vi "printDaqChannel.vi"(8 "error in":errorcluster, 9 "Indent":i32, 10 "TreeRef":refnum<vi>, 11 "baseObject in":refnum<class "IBaseObject.lvclass">) -> (0 "error out":errorcluster, 3 "baseObject out":refnum<class "IBaseObject.lvclass">)   [LabVIEW 2022 SP3, in "openDAQ.lvlib" / "daqUtils.lvlib" / "Tree.lvlib"]
uses:
  Tree.lvlib
  IBaseObject/IBaseObject.lvclass
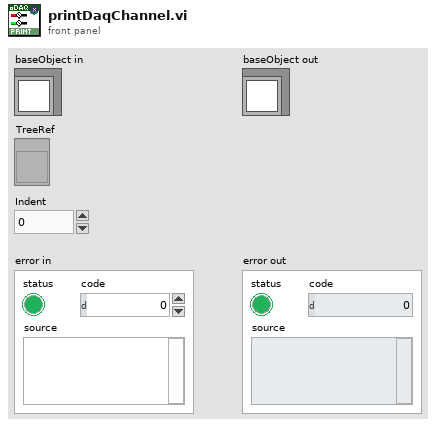
[diagram p1: front panel]
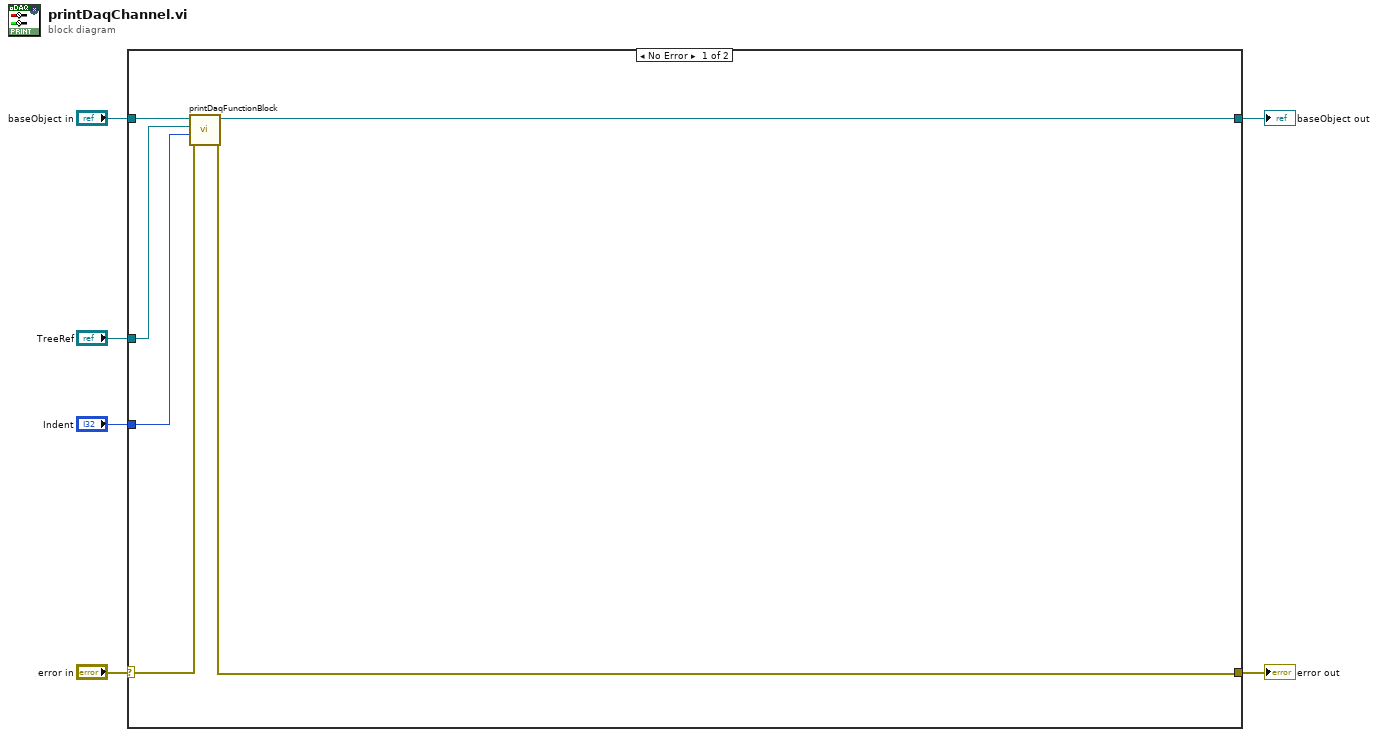
[diagram p0: block diagram]
diagram:
  n1 = case shown="No Error" "error in" {
    selector: "error in" -> [w11 w14]
    tunnel: "baseObject in" -> [w12 w13]
    tunnel: "Indent" -> [w7 _]
    tunnel: "TreeRef" -> [w8 _]
    tunnel: [w9 w14] -> w2
    tunnel: [w10 w13] -> w1
    frame No Error {
      n2 = call "printDaqFunctionBlock.vi"("error in"=w11, "Indent"=w7, "TreeRef"=w8, "baseObject in"=w12) -> ("error out"=w9:errorcluster, "baseObject out"=w10:refnum<class "IBaseObject.lvclass">)  [unwired: 6 in]
    }
    frame Error {
    }
  }
  "error out" <- w2
  "baseObject out" <- w1
